vi "Destroy to Channel.vi"(8 "Error In":errorcluster, 10 "File Info":refnum<class "File Info.lvclass">, 11 "Channel In":refnum<class "Channel.lvclass">) -> (0 "Error Out":errorcluster, 3 "Channel Out":refnum<class "Channel.lvclass">)   [LabVIEW 2018, in "Toolkit.lvlib" / "File Info.lvclass"]
uses:
  File Info.lvclass
  Channel/Channel.lvclass
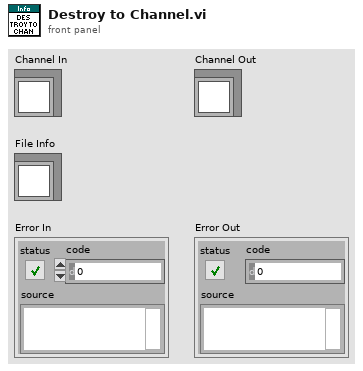
[diagram p1: front panel]
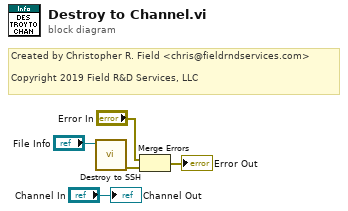
[diagram p0: block diagram]
diagram:
  # "Created by Christopher R. Field <chris@fieldrndservices.com>\n\nCopyright 2019 Field R&D Services, LLC"
  n1 = call "Destroy to SSH.vi"("File Info"="File Info") -> ("Error Out"=w2:errorcluster)  [unwired: 9 in, 1 out]
  n2 = Merge Errors("Error In", w2) -> (→"Error Out":errorcluster)
  "Channel Out" <- "Channel In"
